vi "Get Address DVR.vi"(8 "error in":errorcluster, 11 "class path":path) -> (0 "error out":errorcluster, 3 "DVR Out":refnum<data-value>)   [LabVIEW 2020, in "Address.lvclass"]
uses:
  Address.lvclass
  Address.lvclass/Address.ctl
panel:
  out "Address out":refnum<class "Address.lvclass">
  in  "Address in":refnum<class "Address.lvclass">
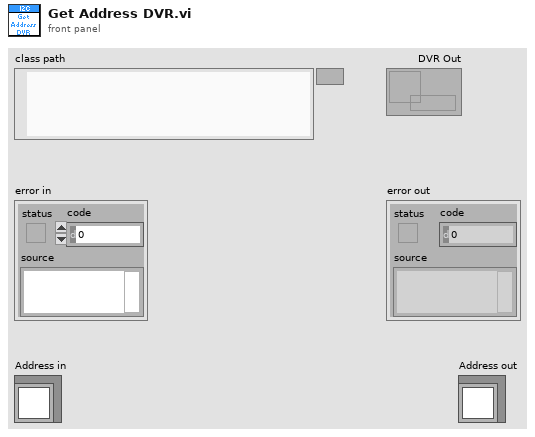
[diagram p1: front panel]
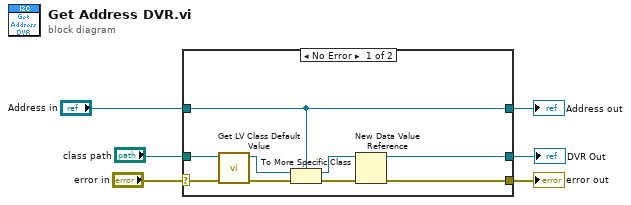
[diagram p0: block diagram]
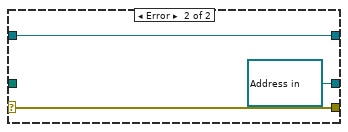
[diagram p2: hidden frame]
diagram:
  n1 = case shown="No Error" "error in" {
    selector: "error in" -> [w15 w18]
    tunnel: [w9 w18] -> w5
    tunnel: [w11 w17] -> w3
    tunnel: "Address in" -> [w11 w17]
    tunnel: "class path" -> [w14 _]
    tunnel: [w7 refnum<data-value> refnum ("data value reference")] -> w1
    frame No Error {
      n2 = call <vilib>:"Get LV Class Default Value.vi"("error in (no error)"=w15, "class path"=w14) -> ("error out"=w13:errorcluster, "object"=w12:refnum<class>)  [unwired: 8 in]
      n3 = To More Specific Class(target class=w11, reference=w12, error in=w13) -> (specific class reference=w8:refnum<class "Address.lvclass">, error out=w10:errorcluster)
      n4 = New Data Value Reference(data value=w8, error in=w10) -> (data value reference=w7:refnum<data-value>, error out=w9:errorcluster)
    }
    frame Error {
    }
  }
  "error out" <- w5
  "Address out" <- w3
  "DVR Out" <- w1
